vi "UART Write Bytes Interval.vi"(6 "IntervalTimeMs":u8, 7 "DataSize":i32, 9 "pWriteData":dbl[](array[numeric])=array[4097 elements], 10 "Channel":u8, 11 "DevHandle":i32) -> (1 "pWriteData out":dbl[](array[numeric]), 3 "function return":i32)   [LabVIEW 2010, in "usb2uart.lvlib"]
doc: "int WINAPI UART_WriteBytesInterval(int DevHandle,unsigned char Channel,unsigned char *pWriteData,int DataSize,unsigned char IntervalTimeMs);"
uses:
  usb2uart.lvlib
  USB2XXX.dll
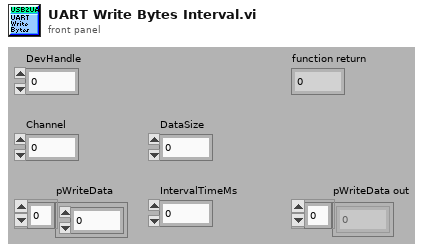
[diagram p1: front panel]
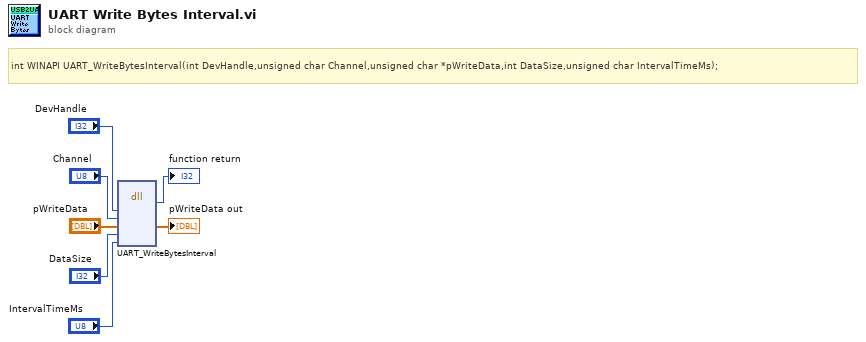
[diagram p0: block diagram]
diagram:
  # "int WINAPI UART_WriteBytesInterval(int DevHandle,unsigned char Channel,unsigned char *pWriteData,int DataSize,unsigned char IntervalTimeMs);"
  n1 = dll-call lib="E:/OtherWork/STM32/USB2XXX_Example/trunk/SDK/api/Labview/USB2XXX.*" fn="UART_WriteBytesInterval"("DevHandle"="DevHandle", "Channel"="Channel", "pWriteData"="pWriteData", "DataSize"="DataSize", "IntervalTimeMs"="IntervalTimeMs") -> (→"function return":i32, "pWriteData"=→"pWriteData out":dbl[])  [unwired: 7 in, 2 out]
